vi "Robot Global Data.vi"() -> ()   [LabVIEW 2017]
doc: "This global VI can contain as many global variables as you need. To create a global variable, place a control on the panel, give it a good name. To read or write to it from a VI, drag the icon to the diagram of that VI. You can also drag from the project. Click on the node to change which global you access. You shouldn't have multiple locations writing to a global or it will cause a race-condition."
uses:
  <vilib>/Rock Robotics/WPI/Camera/WPI_CameraImageSize.ctl
  <vilib>/Rock Robotics/WPI/DriverStation/WPI_DriverStationRobotMode2.ctl
panel:
  in  "Move Hook Arm Down Button":bool
  in  "Move Hook Arm Up Button":bool
  in  "Clear PDP Sticky Fault":bool
  in  "Move Hook Arm":dbl
  in  "Move Hook":dbl
  in  "Move Grabber":dbl
  in  "Move Arm":dbl
  in  "Right Turn Button":bool
  in  "Left Turn Button":bool
  in  "Drive Turn":dbl
  in  "Drive Speed":dbl
  in  "Right Turn Time (ms)":dbl
  in  "Left Turn Time (ms)":dbl
  in  "Rate reduction":dbl
  in  "Min Output(0 to 1)":dbl
  in  "Select Mode":T1(ring)=enum."Exponential"
  in  "n^x(Unbounded)":dbl=2.5 format="%#_13g"
  in  "Sonar Distance":dbl
  in  "Robot Mode":T2
  in  "image size":T3=enum."320x240"
  in  "Enable Vision":bool
  # "Drive Settings"
  # "Joystick 0 Values"
  # "Joystick 1 Values"
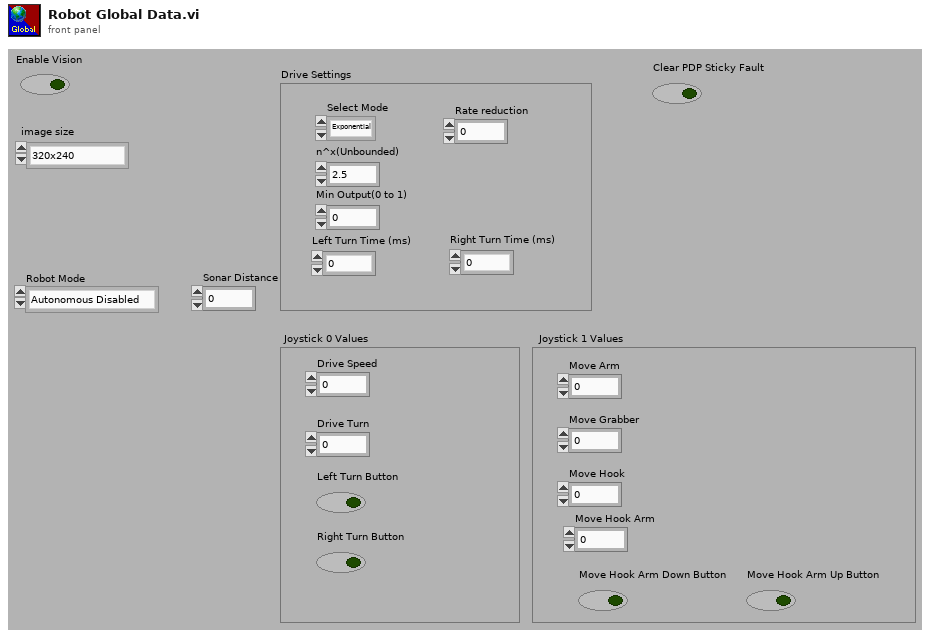
[diagram p1: front panel]
types:
  T1 = enum16{"Normal", "Square", "Square with Rate", "Square Root", "Linear", "Exponential"}
  T2 = typedef "WPI_DriverStationRobotMode2.ctl" = enum16{"Autonomous Disabled", "Autonomous Enabled", "Teleop Disabled", "Teleop Enabled", "Disconnected", "Finish", "Test Disabled", "Test Enabled", "Emergency Stopped"}
  T3 = typedef "WPI_CameraImageSize.ctl" = enum16{"640x480", "320x240", "160x120", "Custom"}
diagram:
